vi "CAN.Initialize.vi"(8 "error in (no error)":errorcluster, 11 "Parameters":T1={"Properties"={"Name"="", "CAN"={"CAN Interface"=enum."CAN0", "Baud Rate"=0, "Diagnostic Protocol"=enum."GMLAN", "Transport Protocol"=enum."ISO TP - Normal Mode", "Transmit ID"=0, "Receive ID"=0, "Transmit Extension"=0, "Receive Extension"=0, "Receive UUDT ID"=0, "Enable Stream"=TRUE, "VW TP Channel ID"=0, "Security"={"Source DLL Path"=path "", "Security Level"=1, "Target DLL Path"=path ""}, "Fill Frame"=FALSE, "Fill Byte"=255, "Termination"=FALSE}, "986x"={"Enable"=FALSE, "RIO Device"=0, "Bitfile"=path ""}, "Reads"=[], "Frames Lookup"=variant, "Writes"=[], "DPIDs"=[], "DPID Lookup"=variant, "DTC descriptor"={"DTC Byte Length"=2, "Status Byte Length"=1, "Add Data Byte Length"=1, "Byte Order"=enum."Motorola"}}, "ChanRefs"={"ToVS.Reads"={"Name"="", "Write to VS Engine FIFO"=refnum, "Pairs"={"Refs"=[], "Values"=[]}}, "ToVS.DTCs"={"Name"="", "Write to VS Engine FIFO"=refnum, "Pairs"={"Refs"=[], "Values"=[]}}, "ToVS.DTCCount"={"Name"="", "Write to VS Engine FIFO"=refnum, "Pairs"={"Refs"=[], "Values"=[]}}, "ToVS.Status"={"Name"="", "Write to VS Engine FIFO"=refnum, "Pairs"={"Refs"=[], "Values"=[]}}, "FromVS.Writes"={"Name"="", "Read from VS Engine FIFO"=refnum, "Pairs"={"Refs"=[], "Values"=[]}}, "Cmds"={"Name"="", "Write to VS Engine FIFO"=refnum, "Read from VS Engine FIFO"=refnum, "Pairs"={"Chan Refs"=[], "Prev. Values"=[]}}}} {"ChanRefs"."Cmds"."Pairs"."Chan Refs" format="%.0x"; "ChanRefs"."FromVS.Writes"."Pairs"."Refs"."Data Reference" format="%.0x"; "ChanRefs"."ToVS.Status"."Pairs"."Refs" format="%.0x"; "ChanRefs"."ToVS.DTCCount"."Pairs"."Refs" format="%.0x"; "ChanRefs"."ToVS.DTCs"."Pairs"."Refs" format="%.0x"; "ChanRefs"."ToVS.Reads"."Pairs"."Refs" format="%.0x"; "Properties"."Writes"."Signals"."Byte Order" items=["Little Endian", "Big Endian"]; "Properties"."Writes"."Signals"."Data Type" items=["Signed", "Unsigned", "IEEE Float"]; "Properties"."CAN"."Fill Byte" format="%.0x"; "Properties"."CAN"."VW TP Channel ID" format="%.0x"; "Properties"."CAN"."Receive UUDT ID" format="%.0x"; "Properties"."CAN"."Receive Extension" format="%.0x"; "Properties"."CAN"."Transmit Extension" format="%.0x"; "Properties"."CAN"."Receive ID" format="%.0x"; "Properties"."CAN"."Transmit ID" format="%.0x"; "Properties"."Reads"."Signals"."Byte Order" items=["Little Endian", "Big Endian"]; "Properties"."Reads"."Signals"."Data Type" items=["Signed", "Unsigned", "IEEE Float"]}) -> (0 "error out":errorcluster, 1 "ADCS Connection":T22, 2 "XNET References":T21, 3 "Parameters":T1={"Properties"={"Name"="", "CAN"={"CAN Interface"=enum."CAN0", "Baud Rate"=0, "Diagnostic Protocol"=enum."GMLAN", "Transport Protocol"=enum."ISO TP - Normal Mode", "Transmit ID"=0, "Receive ID"=0, "Transmit Extension"=0, "Receive Extension"=0, "Receive UUDT ID"=0, "Enable Stream"=TRUE, "VW TP Channel ID"=0, "Security"={"Source DLL Path"=path "", "Security Level"=1, "Target DLL Path"=path ""}, "Fill Frame"=FALSE, "Fill Byte"=255, "Termination"=FALSE}, "986x"={"Enable"=FALSE, "RIO Device"=0, "Bitfile"=path ""}, "Reads"=[], "Frames Lookup"=variant, "Writes"=[], "DPIDs"=[], "DPID Lookup"=variant, "DTC descriptor"={"DTC Byte Length"=2, "Status Byte Length"=1, "Add Data Byte Length"=1, "Byte Order"=enum."Motorola"}}, "ChanRefs"={"ToVS.Reads"={"Name"="", "Write to VS Engine FIFO"=refnum, "Pairs"={"Refs"=[], "Values"=[]}}, "ToVS.DTCs"={"Name"="", "Write to VS Engine FIFO"=refnum, "Pairs"={"Refs"=[], "Values"=[]}}, "ToVS.DTCCount"={"Name"="", "Write to VS Engine FIFO"=refnum, "Pairs"={"Refs"=[], "Values"=[]}}, "ToVS.Status"={"Name"="", "Write to VS Engine FIFO"=refnum, "Pairs"={"Refs"=[], "Values"=[]}}, "FromVS.Writes"={"Name"="", "Read from VS Engine FIFO"=refnum, "Pairs"={"Refs"=[], "Values"=[]}}, "Cmds"={"Name"="", "Write to VS Engine FIFO"=refnum, "Read from VS Engine FIFO"=refnum, "Pairs"={"Chan Refs"=[], "Prev. Values"=[]}}}} {"ChanRefs"."Cmds"."Pairs"."Chan Refs" format="%.0x"; "ChanRefs"."FromVS.Writes"."Pairs"."Refs"."Data Reference" format="%.0x"; "ChanRefs"."ToVS.Status"."Pairs"."Refs" format="%.0x"; "ChanRefs"."ToVS.DTCCount"."Pairs"."Refs" format="%.0x"; "ChanRefs"."ToVS.DTCs"."Pairs"."Refs" format="%.0x"; "ChanRefs"."ToVS.Reads"."Pairs"."Refs" format="%.0x"; "Properties"."Writes"."Signals"."Byte Order" items=["Little Endian", "Big Endian"]; "Properties"."Writes"."Signals"."Data Type" items=["Signed", "Unsigned", "IEEE Float"]; "Properties"."CAN"."Fill Byte" format="%.0x"; "Properties"."CAN"."VW TP Channel ID" format="%.0x"; "Properties"."CAN"."Receive UUDT ID" format="%.0x"; "Properties"."CAN"."Receive Extension" format="%.0x"; "Properties"."CAN"."Transmit Extension" format="%.0x"; "Properties"."CAN"."Receive ID" format="%.0x"; "Properties"."CAN"."Transmit ID" format="%.0x"; "Properties"."Reads"."Signals"."Byte Order" items=["Little Endian", "Big Endian"]; "Properties"."Reads"."Signals"."Data Type" items=["Signed", "Unsigned", "IEEE Float"]})   [LabVIEW 2015, in "Diagnostics Addon Engine.lvlib"]
uses:
  Diagnostics Addon Engine.lvlib
  Types/Engine.State.ctl
  Shared/Types/SysDef.Compile.Properties.ctl
  Shared/Types/CAN.ctl
  Shared/Types/CAN.Interface.ctl
  Shared/Types/Protocol.ctl
  Shared/Types/Transport.ctl
  Shared/Types/Security.ctl
  Shared/Types/986x.ctl
  Shared/Types/Frame.Compile.ctl
  Shared/Types/Type.ctl
  Shared/Types/Signal.ctl
  Shared/Types/DPID.ctl
  Shared/Types/DPID.Rate.ctl
  Shared/Types/DTCDescriptor.ctl
  Types/Engine.Refs.ctl
  Inline Async API/Controls/Write To VS Engine.ctl
  <vilib>/NI Veristand/Custom Device API/Data Reference.ctl
  Inline Async API/Controls/Read From VS Engine.ctl
  <vilib>/NI Veristand/Custom Device API/Block Data Reference.ctl
  Inline Async API/Controls/ReadWrite Data.ctl
  <vilib>/Automotive Diagnostic Command Set/Diagnostic Transport.llb/Diag Reference.ctl
  <vilib>/Automotive Diagnostic Command Set/Diagnostic Transport.llb/Transport Protocol Selector.ctl
  <vilib>/Automotive Diagnostic Command Set/Diagnostic Transport.llb/Diag CAN Frame Log.ctl
  Types/XNET.Refs.ctl
  <vilib>/Automotive Diagnostic Command Set/Diagnostic Transport.llb/Property ID.ctl
  <vilib>/Automotive Diagnostic Command Set/Diagnostic Transport.llb/VWTP Application Type.ctl
  <vilib>/Automotive Diagnostic Command Set/Diagnostic Transport.llb/DoIP OpenType.ctl
  <vilib>/xnet/xnet.llb/XNET Create Session (Frame Input Queued).vi
  <vilib>/addons/Automotive Diagnostic Command Set/NI_Automotive Diagnostic Command Set.lvlib
  <vilib>/NI Veristand/Custom Device Tools/Custom Device Utility Library/Custom Device Utility Library.lvlib
  Shared/Diagnostics Addon Shared.lvlib
  <vilib>/NI Veristand/Custom Device API/Custom Device API.lvlib
  Inline Async API/Inline Async API.lvlib
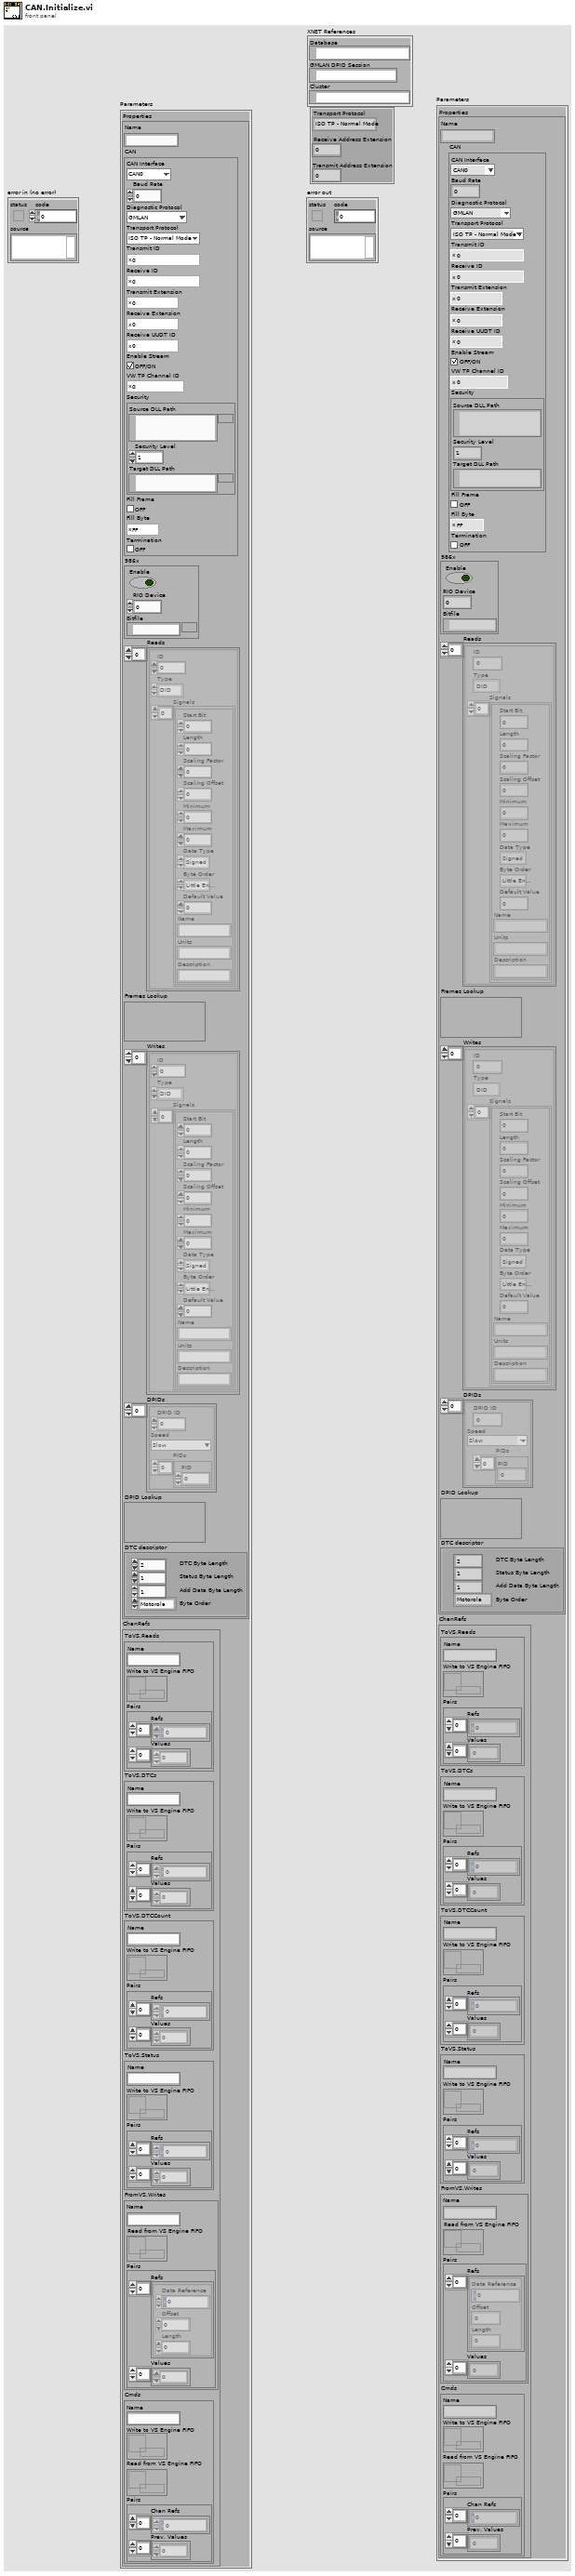
[diagram p1: front panel]
types:
  T1 = typedef "Diagnostics Addon Engine.lvlib/Engine.State.ctl" = cluster{"Properties":T2, "ChanRefs":T15}
  T2 = typedef "Diagnostics Addon Shared.lvlib/SysDef.Compile.Properties.ctl" = cluster{"Name":string, "CAN":T3, "986x":T8, "Reads":T9[], "Frames Lookup":variant, "Writes":T9[], "DPIDs":T12[], "DPID Lookup":variant, "DTC descriptor":T14}
  T3 = typedef "Diagnostics Addon Shared.lvlib/CAN.ctl" = cluster{"CAN Interface":T4, "Baud Rate":u32, "Diagnostic Protocol":T5, "Transport Protocol":T6, "Transmit ID":u32, "Receive ID":u32, "Transmit Extension":u8, "Receive Extension":u8, "Receive UUDT ID":u32, "Enable Stream":bool, "VW TP Channel ID":u32, "Security":T7, "Fill Frame":bool, "Fill Byte":u8, "Termination":bool}
  T4 = typedef "Diagnostics Addon Shared.lvlib/CAN.Interface.ctl" = enum16{"CAN0", "CAN1", "CAN2", "CAN3", "CAN4", "CAN5", "CAN6", "CAN7", "CAN8", "CAN9", "CAN10", "CAN11", "CAN12", "CAN13", "CAN14", "CAN15", "CAN16", "CAN17", "CAN18", "CAN19", "CAN20", "CAN21", "CAN22", "CAN23", "CAN24", "CAN25", "CAN26", "CAN27", "CAN28", "CAN29", "CAN30", "CAN31", "CAN32", "CAN33", "CAN34", "CAN35", "CAN36", "CAN37", "CAN38", "CAN39", "CAN40", "CAN41", "CAN42", "CAN43", "CAN44", "CAN45", "CAN46", "CAN47", "CAN48", "CAN49", "CAN50", "CAN51", "CAN52", "CAN53", "CAN54", "CAN55", "CAN56", "CAN57", "CAN58", "CAN59", "CAN60", "CAN61", "CAN62", "CAN63", "CAN 256 (Virtual)", "CAN 257 (Virtual)"}
  T5 = typedef "Diagnostics Addon Shared.lvlib/Protocol.ctl" = enum16{"GMLAN", "KWP-2000", "UDS"}
  T6 = typedef "Diagnostics Addon Shared.lvlib/Transport.ctl" = enum16{"ISO TP - Normal Mode", "ISO TP - Mixed Mode", "VW TP 2.0", "Diagnostics on IP"}
  T7 = typedef "Diagnostics Addon Shared.lvlib/Security.ctl" = cluster{"Source DLL Path":path, "Security Level":u8, "Target DLL Path":path}
  T8 = typedef "Diagnostics Addon Shared.lvlib/986x.ctl" = cluster{"Enable":bool, "RIO Device":u16, "Bitfile":path}
  T9 = typedef "Diagnostics Addon Shared.lvlib/Frame.Compile.ctl" = cluster{"ID":u32, "Type":T10, "Signals":T11[]}
  T10 = typedef "Diagnostics Addon Shared.lvlib/Type.ctl" = enum16{"DID", "CDID", "PID", "CPID", "Read Memory", "Write Memory", "DTC Control", "IO Cmd", "IO Resp", "Routine Start Cmd", "Routine Start Resp", "Routine Request Cmd", "Routine Request Resp", "Routine Stop Cmd", "Routine Stop Resp"}
  T11 = typedef "Diagnostics Addon Shared.lvlib/Signal.ctl" = cluster{"Start Bit":u8, "Length":u8, "Scaling Factor":dbl, "Scaling Offset":dbl, "Minimum":dbl, "Maximum":dbl, "Data Type":u32, "Byte Order":u32, "Default Value":dbl, "Name":string, "Units":string, "Description":string}
  T12 = typedef "Diagnostics Addon Shared.lvlib/DPID.ctl" = cluster{"DPID ID":u8, "Speed":T13, "PIDs":u16[]}
  T13 = typedef "Diagnostics Addon Shared.lvlib/DPID.Rate.ctl" = enum16{"Slow", "Medium", "Fast"}
  T14 = typedef "Diagnostics Addon Shared.lvlib/DTCDescriptor.ctl" = cluster{"DTC Byte Length":i32, "Status Byte Length":i32, "Add Data Byte Length":i32, "Byte Order":enum16{"Motorola", "Intel"}}
  T15 = typedef "Diagnostics Addon Engine.lvlib/Engine.Refs.ctl" = cluster{"ToVS.Reads":T16, "ToVS.DTCs":T16, "ToVS.DTCCount":T16, "ToVS.Status":T16, "FromVS.Writes":T18, "Cmds":T20}
  T16 = typedef "Diagnostics Addon Engine.lvlib/Inline Async API.lvlib/Write To VS Engine.ctl" = cluster{"Name":string, "Write to VS Engine FIFO":refnum<k33>, "Pairs":cluster{"Refs":T17[], "Values":dbl[]}}
  T17 = typedef "Custom Device API.lvlib/Data Reference.ctl" = i32
  T18 = typedef "Diagnostics Addon Engine.lvlib/Inline Async API.lvlib/Read From VS Engine.ctl" = cluster{"Name":string, "Read from VS Engine FIFO":refnum<k33>, "Pairs":cluster{"Refs":T19[], "Values":dbl[]}}
  T19 = typedef "Custom Device API.lvlib/Block Data Reference.ctl" = cluster{"Data Reference":T17, "Offset":u64, "Length":u64}
  T20 = typedef "Diagnostics Addon Engine.lvlib/Inline Async API.lvlib/ReadWrite Data.ctl" = cluster{"Name":string, "Write to VS Engine FIFO":refnum<k33>, "Read from VS Engine FIFO":refnum<k33>, "Pairs":cluster{"Chan Refs":T17[], "Prev. Values":dbl[]}}
  T21 = typedef "Diagnostics Addon Engine.lvlib/XNET.Refs.ctl" = cluster{"Database":refnum<k21>, "GMLAN DPID Session":refnum<k21>, "Cluster":refnum<k21>}
  T22 = typedef "NI_Automotive Diagnostic Command Set.lvlib/Diag Reference.ctl" = cluster{"Diag CAN Handle":u32, "Transport Protocol":T23, "Receive Address Extension":u8, "Transmit Address Extension":u8, "Receive CAN Id":u32, "Transmit CAN Id":u32, "Diag CAN Queue":refnum<queue>, "Log Frames ?":bool, "My TP Address":u8, "Other TP Address":u8, "T1":u16, "T2":u16, "T3":u16, "T4":u16, "Tx SN":u8, "Block Size":u8, "Rx SN":u8, "VW TP Initialized?":bool, "Tx block no":u8, "baud rate":u32, "Interface":string, "Channel Diag CAN Handle":u32, "UDP Connection ID":refnum<k16>, "TCP Connection ID":refnum<k5>, "Target IP Addr":u32, "Source Address":u16, "Target Address":u16, "Send Header NACK?":bool, "DLL Handle":u32, "NAD":u8, "Time Stamp read first":dbl, "Time Stamp read last":dbl, "Time Stamp write first":dbl, "Time Stamp write last":dbl, "Time Stamp write":dbl, "Time Stamp read":dbl}
  T23 = typedef "NI_Automotive Diagnostic Command Set.lvlib/Transport Protocol Selector.ctl" = enum16{"ISO TP - Normal Mode", "ISO TP - Mixed Mode", "VW TP 2.0", "Diagnostics on IP", "ISO TP LIN"}
  T24 = typedef "NI_Automotive Diagnostic Command Set.lvlib/Property ID.ctl" = enum16{"Timeout Diag Command", "Timeout FC (Bs)", "Timeout CF (Cr)", "Receive Block Size (BS)", "Wait Time CF (STmin)", "Max Wait Frames (N_WFTmax)", "Wait Frames to Send (N_WAIT)", "Time between Waits (T_W)", "Fill CAN Frames", "Fill Byte", "Invalid Response as Error", "Max RspPending Count", "VWTP Command Timeout", "STmin", "P2min", "Termination"}
  T25 = typedef "NI_Automotive Diagnostic Command Set.lvlib/VWTP Application Type.ctl" = u8
  T26 = typedef "NI_Automotive Diagnostic Command Set.lvlib/DoIP OpenType.ctl" = u16
  T27 = typedef "NI_Automotive Diagnostic Command Set.lvlib/DoIP Vehicle ID Cluster.ctl" = cluster{"VIN":string, "Source Address":u16, "EID":u8[], "GID":u8[], "IP Address":string}
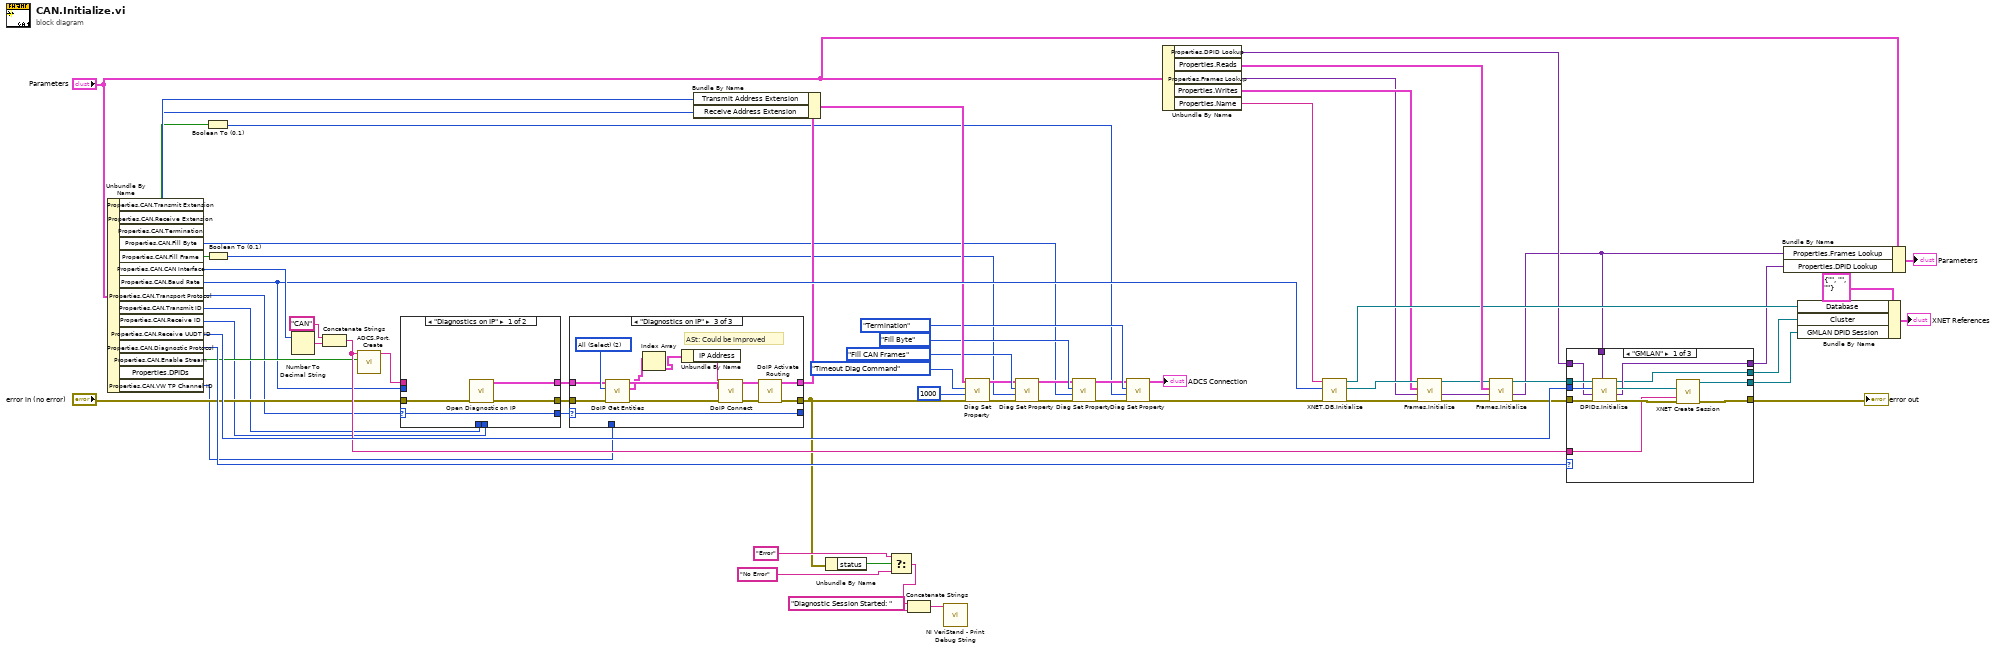
[diagram p0: block diagram]
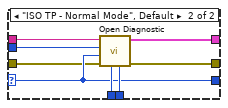
[diagram p2: hidden frame]
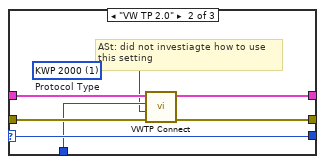
[diagram p4: hidden frame]
diagram:
  n1 = Unbundle By Name("Parameters") -> ("Properties.CAN.Transmit Extension"=w65:u8, "Properties.CAN.Receive Extension"=w64:u8, "Properties.CAN.Termination"=w15:bool, "Properties.CAN.Fill Byte"=w17:u8, "Properties.CAN.Fill Frame"=w16:bool, "Properties.CAN.CAN Interface"=w68:T4, "Properties.CAN.Baud Rate"=w37:u32, "Properties.CAN.Transport Protocol"=w40:T6, "Properties.CAN.Transmit ID"=w36:u32, "Properties.CAN.Receive ID"=w35:u32, "Properties.CAN.Receive UUDT ID"=w55:u32, "Properties.CAN.Diagnostic Protocol"=w54:T5, "Properties.CAN.Enable Stream"=w49:bool, "Properties.CAN.VW TP Channel ID"=w30:u32)  [unwired: 1 out]
  n2 = Boolean To (0,1)(Boolean=w15) -> (0, 1=w14:i16)
  n3 = Boolean To (0,1)(Boolean=w16) -> (0, 1=w13:i16)
  n4 = Number To Decimal String(number=w68) -> (decimal integer string=w67:string)  [unwired: 1 in]
  n5 = Concatenate Strings("CAN" ("string"), w67) -> (w50:string)
  n6 = call "ADCS.Port.Create.vi"("Enable Stream"=w49, "CAN port"=w50) -> ("CAN port out"=w38:string)  [unwired: 9 in]
  n7 = case shown="\"Diagnostics on IP\"" w40 {
    selector: w40 -> [w72 w74]
    tunnel: w36 -> [_ w80]
    tunnel: w37 -> [_ w79]
    tunnel: w35 -> [_ w78]
    tunnel: [w70 w77] -> w34
    tunnel: [w71 w76] -> w32
    tunnel: w38 -> [_ w75]
    tunnel: [w72 w74] -> w39
    tunnel: "error in (no error)" -> [w69 w73]
    frame "Diagnostics on IP" {
      n8 = call <vilib>:"Open Diagnostic on IP.vi"("error in (no error)"=w69) -> ("error out"=w71:errorcluster, "Diag reference out"=w70:T22)  [unwired: 1 in, 8 out]
    }
    frame "ISO TP - Normal Mode", Default {
      n9 = call <vilib>:"Open Diagnostic.vi"("Receive ID"=w78, "Transmit ID"=w80, "error in (no error)"=w73, "Transport Protocol"=w74, "Baud Rate"=w79, "CAN Interface"=w75) -> ("error out"=w76:errorcluster, "diag ref out"=w77:T22)  [unwired: 4 out]
    }
  }
  n10 = case shown="\"Diagnostics on IP\"" w39 {
    selector: w39 -> [w83 w88 w93]
    tunnel: [w82 w90 w96] -> w33
    tunnel: [w81 w89 w94] -> w31
    tunnel: [w83 w88 w93] -> _
    tunnel: w34 -> [w82 w87 w92]
    tunnel: w32 -> [w81 w86 w91]
    tunnel: w30 -> [_ w85 _]
    frame "ISO TP - Normal Mode", Default {
    }
    frame "VW TP 2.0" {
      w84 = T25 1 items=["KWP 2000"=1, "KS Type 010C"=2, "Infotainment communication"=16, "Application protocol"=32, "WFS/WIV"=33]  # Protocol Type
      # "ASt: did not investiagte how to use\nthis setting"
      n11 = call <vilib>:"VWTP Connect.vi"("error in"=w86, "application type"=w84, "channel ID"=w85, "diag ref in"=w87) -> ("error out"=w89:errorcluster, "diag ref out"=w90:T22)  [unwired: 6 out]
    }
    frame "Diagnostics on IP" {
      w103 = T26 2 items=["VIN", "EID", "All (Select)"] ("DoIP Open Type")
      # "ASt: Could be improved"
      n12 = call <vilib>:"DoIP Get Entities.vi"("error in (no error)"=w91, "DoIP Open Type"=w103, "Diag reference in"=w92) -> ("error out"=w100:errorcluster, "DoIP entities"=w99:T27[], "Diag reference out"=w101:T22)  [unwired: 1 in, 5 out]
      n13 = Index Array(array=w99) -> (element=w98:T27)  [unwired: 1 in]
      n14 = Unbundle By Name(w98) -> ("IP Address"=w97:string)
      n15 = call <vilib>:"DoIP Connect.vi"("error in (no error)"=w100, "address"=w97, "Diag Reference in"=w101) -> ("error out"=w95:errorcluster, "Diag reference out"=w102:T22)  [unwired: 2 in, 5 out]
      n16 = call <vilib>:"DoIP Activate Routing.vi"("error in (no error)"=w95, "Diag reference in"=w102) -> ("error out"=w94:errorcluster, "Diag reference out"=w96:T22)  [unwired: 2 in, 6 out]
    }
  }
  n17 = Bundle By Name(cluster=w33, "Transmit Address Extension"=w65, "Receive Address Extension"=w64) -> (w29:T22)
  n18 = Unbundle By Name(w31) -> ("status"=w46:bool)
  n19 = Select(t="Error" ("string"), s=w46, f="No Error" ("string")) -> (s? t:f=w43:string)
  n20 = Concatenate Strings("Diagnostic Session Started: " ("string"), w43) -> (w42:string)
  n21 = call <vilib>:"NI VeriStand - Print Debug String.vi"("Message"=w42) -> ()  [unwired: 10 in, 1 out]
  n22 = call <vilib>:"Diag Set Property.vi"("error in (no error)"=w31, "property value"=u32 1000, "property ID"=Property_ID."Timeout Diag Command", "diag ref in"=w29) -> ("error out"=w26:errorcluster, "diag ref out"=w21:T22)  [unwired: 6 in]
  n23 = call <vilib>:"Diag Set Property.vi"("error in (no error)"=w26, "property value"=w13, "property ID"=Property_ID."Fill CAN Frames", "diag ref in"=w21) -> ("error out"=w28:errorcluster, "diag ref out"=w20:T22)  [unwired: 6 in]
  n24 = call <vilib>:"Diag Set Property.vi"("error in (no error)"=w28, "property value"=w17, "property ID"=Property_ID."Fill Byte", "diag ref in"=w20) -> ("error out"=w27:errorcluster, "diag ref out"=w19:T22)  [unwired: 6 in]
  n25 = call <vilib>:"Diag Set Property.vi"("error in (no error)"=w27, "property value"=w14, "property ID"=Property_ID."Termination", "diag ref in"=w19) -> ("error out"=w25:errorcluster, "diag ref out"=→"ADCS Connection":T22)  [unwired: 6 in]
  n26 = Unbundle By Name("Parameters") -> ("Properties.DPID Lookup"=w52:variant, "Properties.Reads"=w58:T9[], "Properties.Frames Lookup"=w2:variant, "Properties.Writes"=w4:T9[], "Properties.Name"=w8:string)
  n27 = call "XNET.DB.Initialize.vi"("error in (no error)"=w25, "Baud Rate"=w37, "Addon Name"=w8) -> ("error out"=w5:errorcluster, "Cluster"=w7:refnum<k21>, "XNET Database"=w57:refnum<k21>)  [unwired: 6 in]
  n28 = call "Frames.Initialize.vi"("error in"=w5, "Lookup"=w2, "Frames"=w4, "Cluster In"=w7) -> ("error out"=w3:errorcluster, "Lookup"=w1:variant, "Cluster Out"=w6:refnum<k21>)  [unwired: 5 in]
  n29 = call "Frames.Initialize.vi"("error in"=w3, "Lookup"=w1, "Frames"=w58, "Cluster In"=w6) -> ("error out"=w12:errorcluster, "Lookup"=w9:variant, "Cluster Out"=w11:refnum<k21>)  [unwired: 5 in]
  n30 = case shown="\"GMLAN\"" w54 {
    tunnel: w12 -> [w113 w118 w121]
    tunnel: [w105 w118 w121] -> w56
    tunnel: w50 -> [w112 _ _]
    tunnel: w11 -> [w111 w116 w119]
    tunnel: w55 -> [w110 _ _]
    tunnel: [w109 _ _] -> w53
    tunnel: w9 -> [w108 _ _]
    tunnel: w52 -> [w107 w117 w120]
    tunnel: [w106 w117 w120] -> w51
    tunnel: [w104 w116 w119] -> w48
    frame "GMLAN" {
      n31 = call "DPIDs.Initialize.vi"("Read Lookup"=w108, "error in"=w113, "DPID Lookup"=w107, "UUDT Receive ID"=w110, "cluster in"=w111) -> ("error out"=w114:errorcluster, "DPID Lookup Out"=w106:variant, "GMLAN DPID Session"=w115:refnum<k21>, "Cluster Out"=w104:refnum<k21>)  [unwired: 3 in]
      n32 = call-poly <vilib>:"XNET Create Session.vi"("frame"=w115, "interface"=w112, "error in (no error)"=w114) -> ("session out"=w109:refnum<k21>, "error out"=w105:errorcluster)  [unwired: 11 out]
    }
    frame "KWP-2000" {
    }
    frame "UDS" {
    }
  }
  "error out" <- w56
  n33 = Bundle By Name(cluster="Parameters", "Properties.Frames Lookup"=w9, "Properties.DPID Lookup"=w51) -> (→"Parameters":T1)
  n34 = Bundle By Name(cluster=T21 {"Database"="", "GMLAN DPID Session"="", "Cluster"=""}, "Database"=w57, "Cluster"=w48, "GMLAN DPID Session"=w53) -> (→"XNET References":T21)
